vi "Test_baseline_subVIs.vi"() -> ()   [LabVIEW 2013]
uses:
  Sum_array_for_avg_baseline.ctl
  Converter_baseline_indicator.ctl
panel:
  out "baselines for evaluation":dbl[](array[numeric])
  out "baselines for selected unit":string[](array[string])
  in  "From unit #":i32
  out "error out":errorcluster
  in  "error in (no error)":errorcluster
  out "Baselines per unit":T1
  out "Sum array 3":T2
  out "Sum array":T2
  in  "Data in (11vals)":dbl[](array[numeric])
  in  "Data from unit":i32
  # "from baseline per unit indicator, get one column indexed for use to equation"
  # "useless because calculator subvi uses double"
  # "from average array, get one column indexed for use to equation"
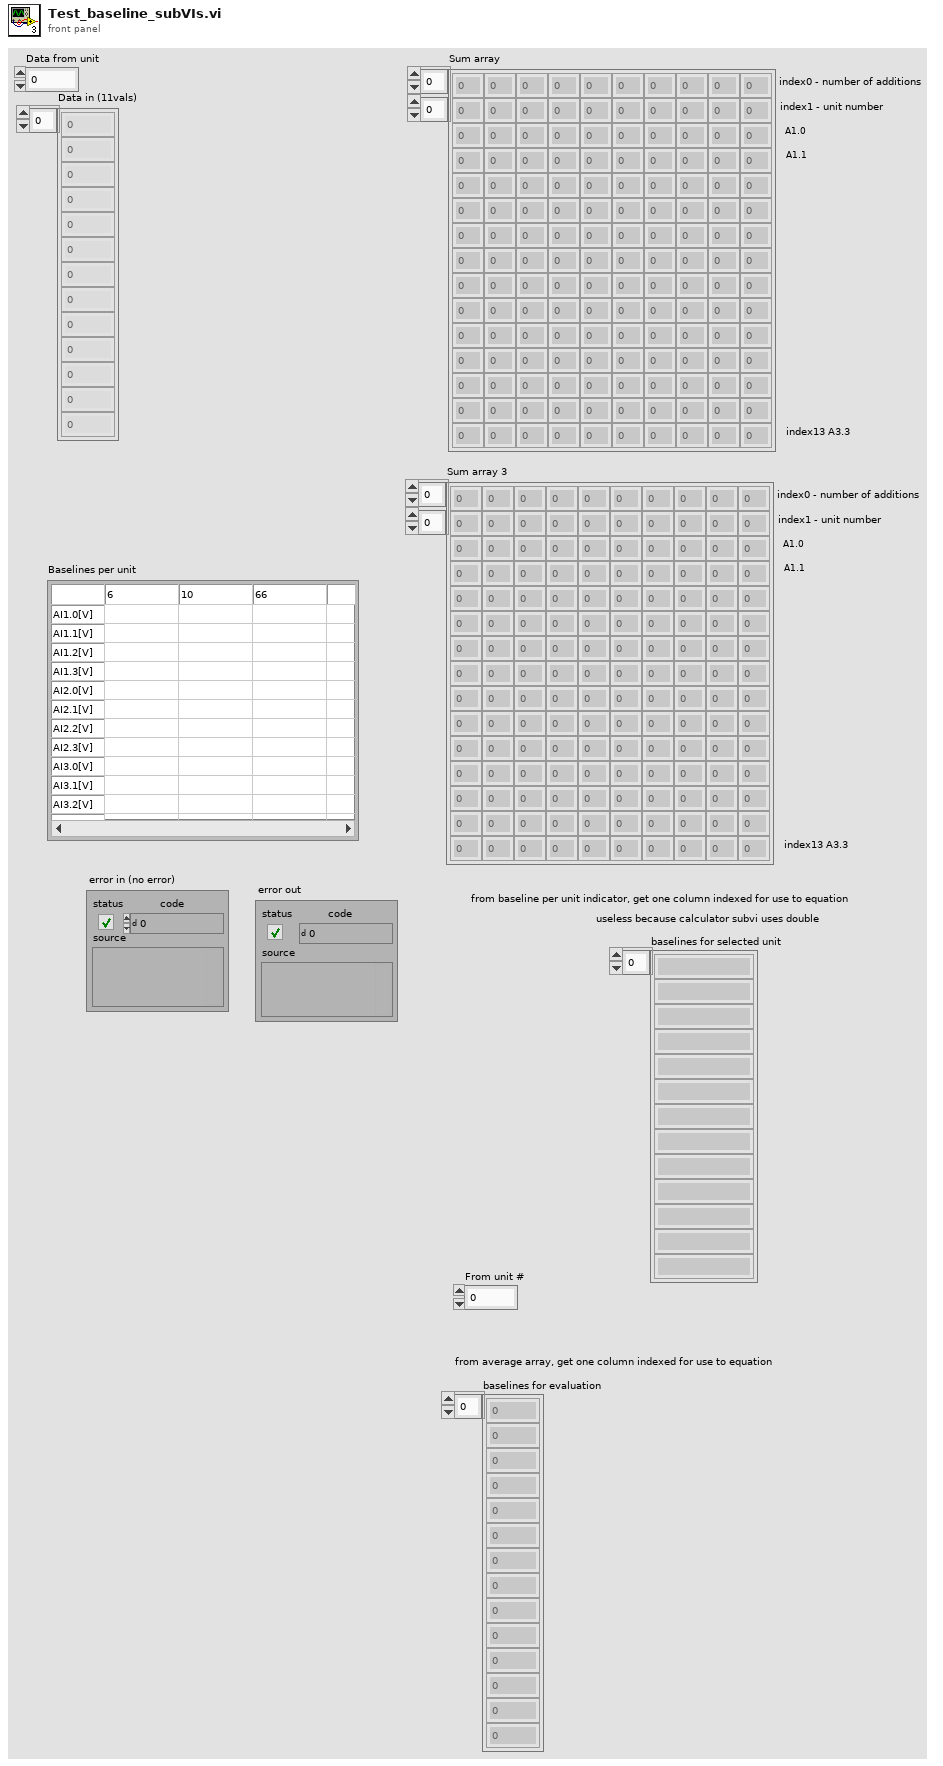
[diagram p1: front panel]
types:
  T1 = typedef "Converter_baseline_indicator.ctl" = string[][]
  T2 = typedef "Sum_array_for_avg_baseline.ctl" = dbl[][]
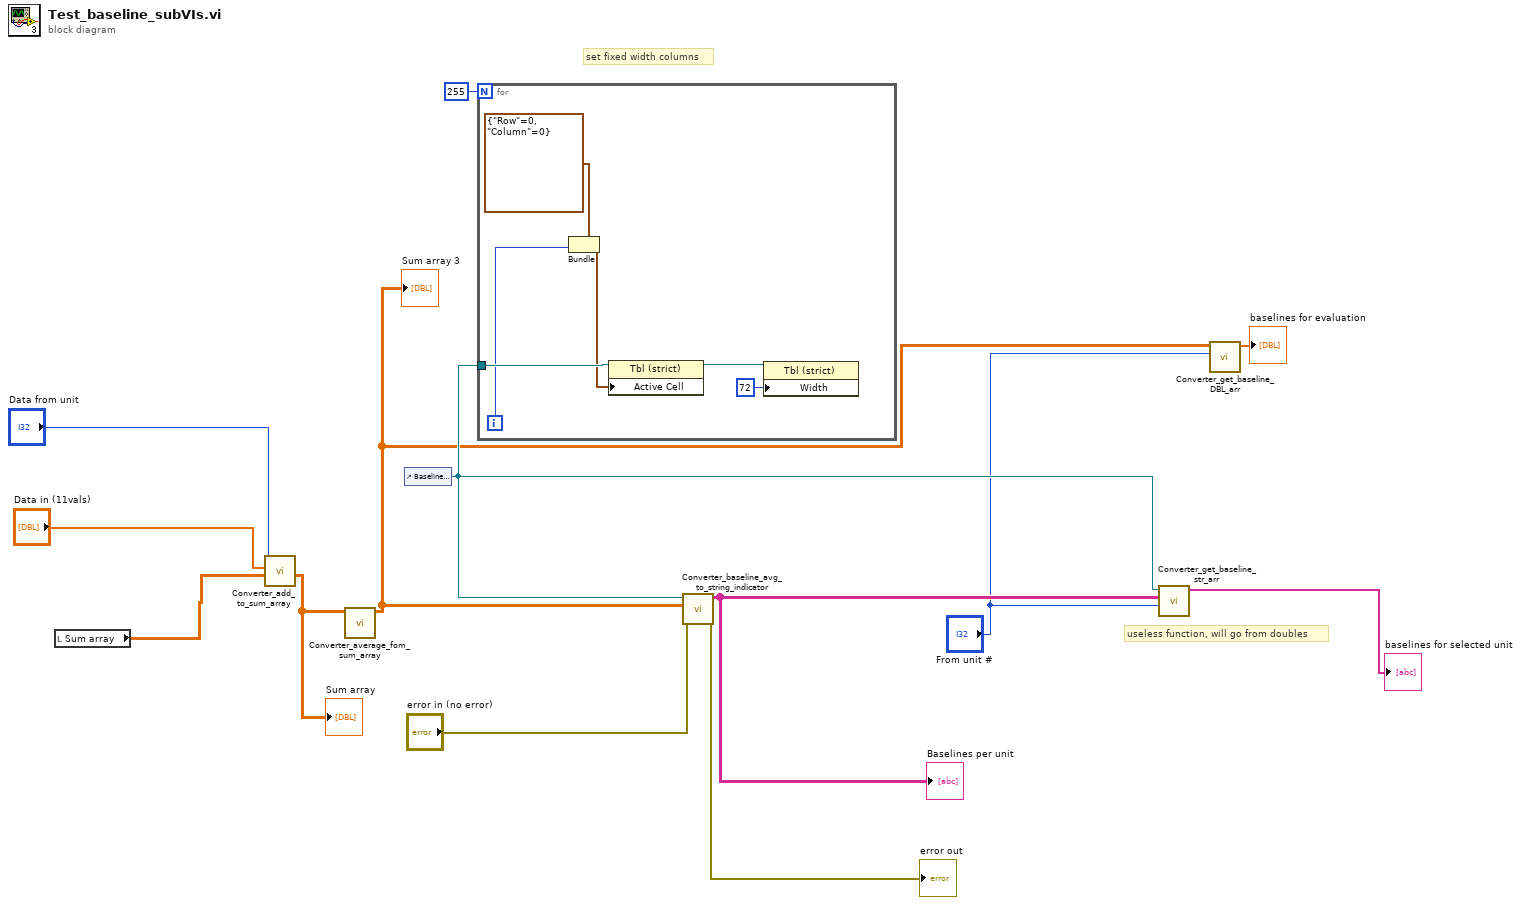
[diagram p0: block diagram]
diagram:
  # "useless function, will go from doubles"
  # "set fixed width columns"
  n1 = local read "Sum array"() -> (w11:T2)
  n2 = call "Converter_add_to_sum_array.vi"("Sum array in"=w11, "Data in (11vals)"="Data in (11vals)", "Data from unit"="Data from unit") -> ("Sum array"=w10:T2)  [unwired: 8 in]
  "Sum array" <- w10
  n3 = call "Converter_average_fom_sum_array.vi"("Sum array in"=w10) -> ("Average array out"=w2:dbl[][])  [unwired: 10 in]
  "Sum array 3" <- w2
  n4 = control-ref of="Baselines per unit"() -> (w6:refnum<vi>)
  n5 = for {
    N: 255 -> [_]
    tunnel: w6 -> [w18]
    i -> [w15]
    n6 = Bundle(cluster=cluster{"Row":i32, "Column":i32} {"Row"=0, "Column"=0}, "Column"=w15) -> (w14:cluster{"Row":i32, "Column":i32})  [unwired: 1 in]
    n7 = property class="Tbl (strict)"(reference=w18, "Active Cell"=w14) -> (reference out=w17:refnum<vi>)  [unwired: 1 in, 1 out]
    n8 = property class="Tbl (strict)"(reference=w17, "Width"=u32 72 ("Active Cell:Cell Size:Width")) -> ()  [unwired: 1 in, 2 out]
  }
  n9 = call "Converter_baseline_avg_to_string_indicator.vi"("error in (no error)"="error in (no error)", "Average array in"=w2, "Ref of baseline indicator"=w6) -> ("error out"=→"error out":errorcluster, "Baselines per unit"=w5:T1)  [unwired: 7 in]
  "Baselines per unit" <- w5
  n10 = call "Converter_get_baseline_str_arr.vi"("From unit #"="From unit #", "Baselines per unit in"=w5, "Table in"=w6) -> ("Baselines per unit out"=→"baselines for selected unit":string[])  [unwired: 8 in]
  n11 = call "Converter_get_baseline_DBL_arr.vi"("From unit #"="From unit #", "Average array in"=w2) -> ("baselines for evaluation"=→"baselines for evaluation":dbl[])  [unwired: 9 in]
